vi "M.vi"(1 "a":ext, 2 "fi[rad]":ext, 3 "e^2":ext) -> (0 "M":ext)   [LabVIEW 2012, in "Biblioteka moduł map v3.lvlib" / "Konwersja wsp.lvlib" / "UTM.lvlib" / "Konwersja z UTM na wsp geograficzne.lvlib"]
uses:
  Konwersja z UTM na wsp geograficzne.lvlib
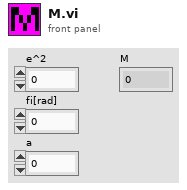
[diagram p1: front panel]
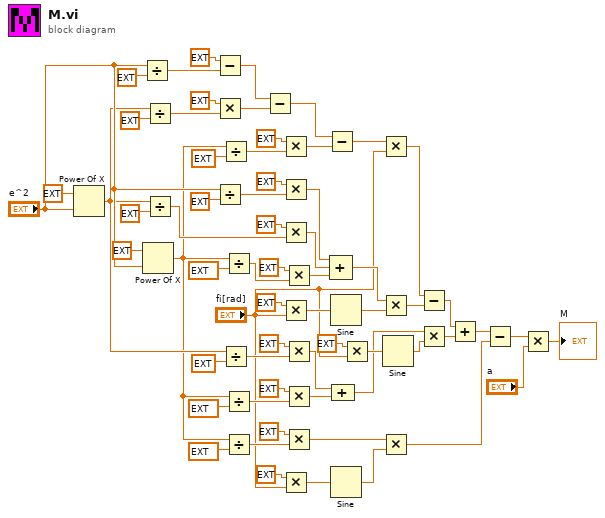
[diagram p0: block diagram]
diagram:
  n1 = Power Of X(1:"e^2", 2:ext 2.0 ("y")) -> (0:w17:ext)
  n2 = Divide(x="e^2", y=ext 4.0) -> (x/y=w59:ext)
  n3 = Power Of X(1:"e^2", 2:ext 3.0 ("y")) -> (0:w10:ext)
  n4 = Divide(x=w17, y=ext 64.0) -> (x/y=w56:ext)
  n5 = Divide(x=w17, y=ext 32.0) -> (x/y=w41:ext)
  n6 = Subtract(x=ext 1.0, y=w59) -> (x-y=w60:ext)
  n7 = Multiply(x=ext 3.0, y=w56) -> (x*y=w57:ext)
  n8 = Divide(x="e^2", y=ext 8.0) -> (x/y=w46:ext)
  n9 = Divide(x=w10, y=ext 256.0) -> (x/y=w52:ext)
  n10 = Divide(x=w17, y=ext 256.0) -> (x/y=w19:ext)
  n11 = Divide(x=w10, y=ext 1024.0) -> (x/y=w38:ext)
  n12 = Divide(x=w10, y=ext 1024.0) -> (x/y=w22:ext)
  n13 = Divide(x=w10, y=ext 3072.0) -> (x/y=w12:ext)
  n14 = Subtract(x=w60, y=w57) -> (x-y=w54:ext)
  n15 = Multiply(x=ext 5.0, y=w52) -> (x*y=w50:ext)
  n16 = Multiply(x=ext 3.0, y=w46) -> (x*y=w43:ext)
  n17 = Multiply(x=ext 3.0, y=w41) -> (x*y=w36:ext)
  n18 = Multiply(x=ext 2.0, y="fi[rad]") -> (x*y=w31:ext)
  n19 = Multiply(x=ext 6.0, y="fi[rad]") -> (x*y=w9:ext)
  n20 = Multiply(x=ext 45.0, y=w38) -> (x*y=w35:ext)
  n21 = Multiply(x=ext 15.0, y=w19) -> (x*y=w24:ext)
  n22 = Multiply(x=ext 45.0, y=w22) -> (x*y=w25:ext)
  n23 = Multiply(x=ext 35.0, y=w12) -> (x*y=w6:ext)
  n24 = Subtract(x=w54, y=w50) -> (x-y=w49:ext)
  n25 = Compound Arithmetic op=ADD(w43, w36, w35) -> (w34:ext)
  n26 = Sine(x=w31) -> (sin(x)=w33:ext)
  n27 = Sine(x=w9) -> (sin(x)=w5:ext)
  n28 = Compound Arithmetic op=ADD(w24, w25) -> (w26:ext)
  n29 = Multiply(x=ext 4.0, y="fi[rad]") -> (x*y=w28:ext)
  n30 = Multiply(x=w49, y="fi[rad]") -> (x*y=w48:ext)
  n31 = Multiply(x=w34, y=w33) -> (x*y=w32:ext)
  n32 = Multiply(x=w6, y=w5) -> (x*y=w4:ext)
  n33 = Sine(x=w28) -> (sin(x)=w27:ext)
  n34 = Subtract(x=w48, y=w32) -> (x-y=w15:ext)
  n35 = Multiply(x=w26, y=w27) -> (x*y=w16:ext)
  n36 = Add(x=w15, y=w16) -> (x+y=w14:ext)
  n37 = Subtract(x=w14, y=w4) -> (x-y=w3:ext)
  n38 = Multiply(x=w3, y="a") -> (x*y=→"M":ext)
